vi "SaveData.vi"(0 "Plain Text Logging in":refnum<class "Plain Text Logging.lvclass">, 1 "Path Control":path, 2 "Signal":dbl[](graph), 3 "error in (no error)":errorcluster) -> (7 "Plain Text Logging out":refnum<class "Plain Text Logging.lvclass">, 10 "error out":errorcluster)   [LabVIEW 2020, in "Plain Text Logging.lvlib" / "Plain Text Logging.lvclass"]
uses:
  Plain Text Logging.lvclass
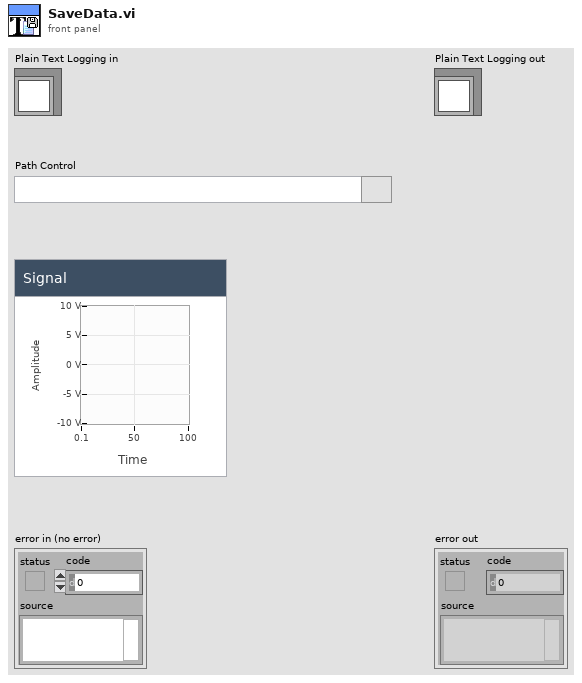
[diagram p1: front panel]
types:
  T1 = enum16{"open", "replace", "create", "open or create", "replace or create", "replace or create with confirmation"}
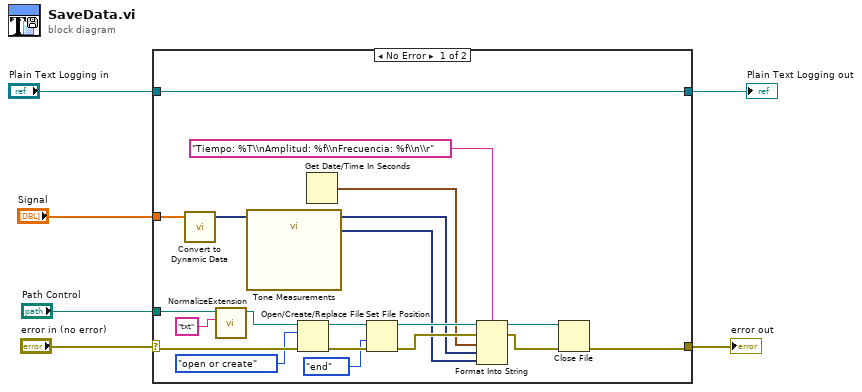
[diagram p0: block diagram]
diagram:
  n1 = case shown="No Error" "error in (no error)" {
    selector: "error in (no error)" -> [w23 w27]
    tunnel: "Plain Text Logging in" -> [w26 w28]
    tunnel: [w26 w28] -> w4
    tunnel: [w7 w27] -> w3
    tunnel: "Path Control" -> [w25 _]
    tunnel: "Signal" -> [w15 _]
    frame No Error {
      n2 = call "Convert to Dynamic Data"("Array"=w15) -> ("Dynamic Data Type"=w14:dynamicdata)  [unwired: 3 in]
      n3 = call "NormalizeExtension.vi"("Extension"="txt", "Path in"=w25) -> ("Path out"=w22:path)  [unwired: 9 in]
      n4 = call "Tone Measurements"("Signals"=w14) -> ("Frequency"=w11:dynamicdata, "Amplitude"=w12:dynamicdata)  [unwired: 8 in, 1 out]
      n5 = Open/Create/Replace File(file path (use dialog)=w22, error in=w23, operation (0:open)=T1."open or create") -> (refnum out=w20:refnum<file>, error out=w19:errorcluster)  [unwired: 3 in, 1 out]
      n6 = Get Date/Time In Seconds() -> (seconds since 1Jan1904=w13:timestamp)
      n7 = Set File Position(refnum=w20, from (0:start)=enum16{"start", "end", "current"}."end", error in=w19) -> (refnum out=w17:refnum<file>, error out=w16:errorcluster)  [unwired: 1 in]
      n8 = Format Into String(format string="Tiempo: %T\\nAmplitud: %f\\nFrecuencia: %f\\n\\r", initial string=w17, error in=w16, w13, w12, w11) -> (resulting string=w9:refnum<file>, error out=w8:errorcluster)
      n9 = Close File(refnum=w9, error in=w8) -> (error out=w7:errorcluster)  [unwired: 1 out]
    }
    frame Error {
    }
  }
  "error out" <- w3
  "Plain Text Logging out" <- w4
